vi "listen connection LV15.vi"(8 "Bool Refnum":refnum<vi>, 10 "service name":string="192.168.1.10") -> (1 "Numeric 2":i32, 2 "Boolean 3":bool, 3 "data out":string)   [LabVIEW 2020]
uses:
  Galobal variable_TI.vi
panel:
  out "length":i32
  out "String":string
  out "error out 3":errorcluster
  # "1,3.644,3.358,7.44,7.546"
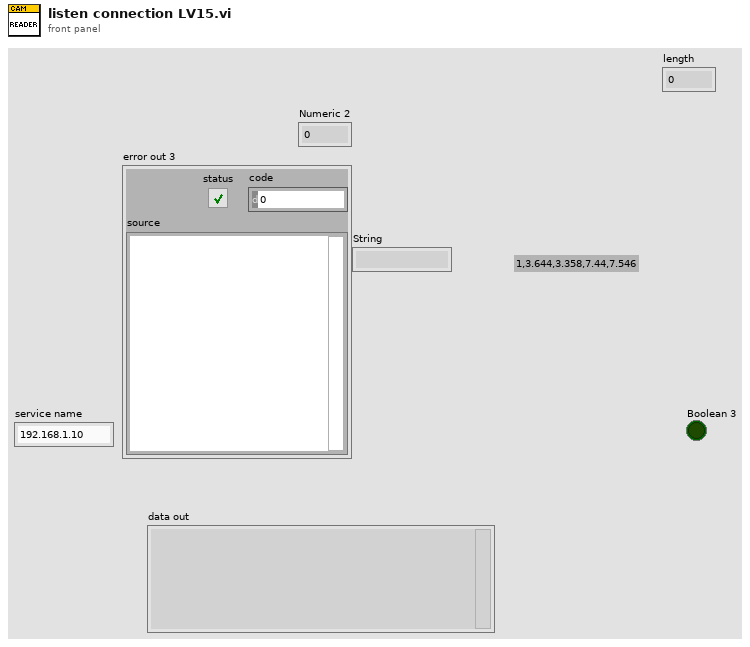
[diagram p1: front panel]
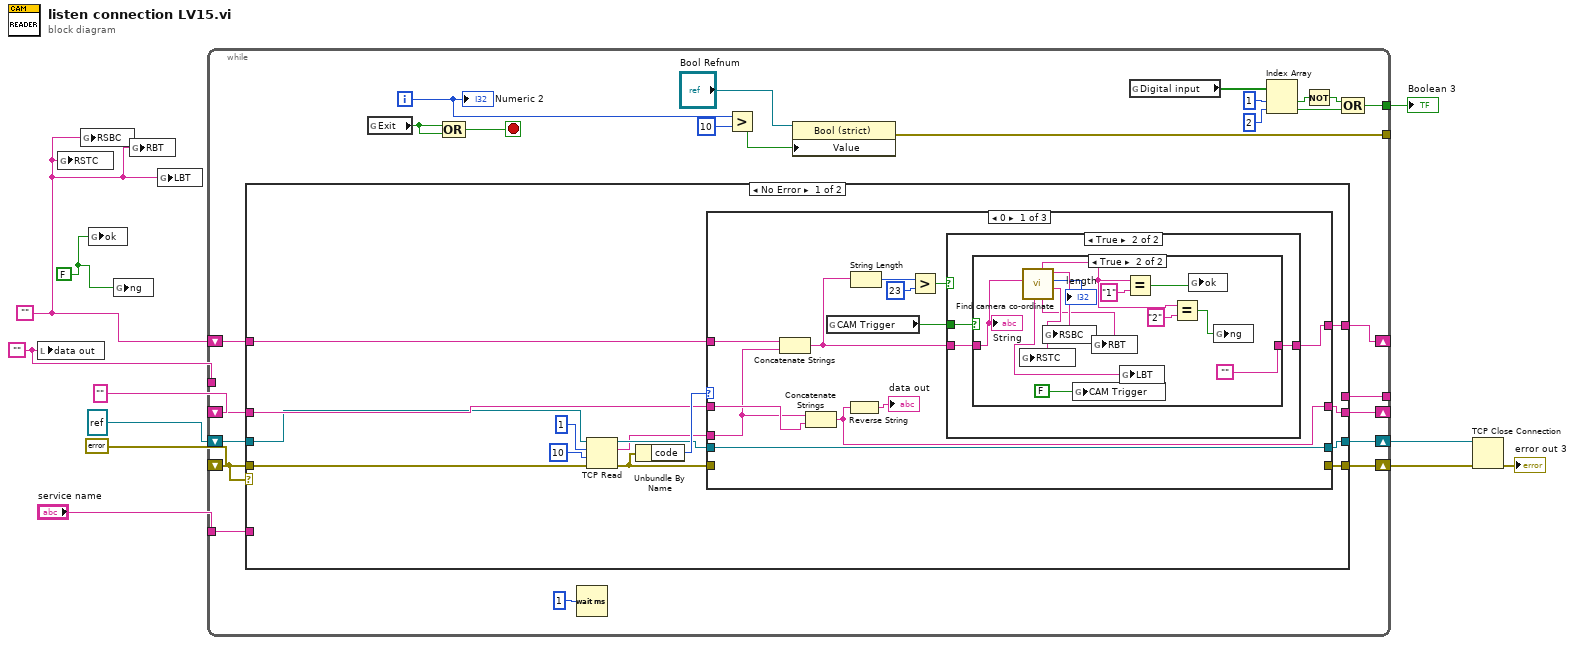
[diagram p0: block diagram]
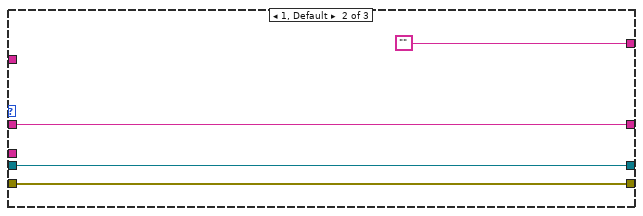
[diagram p4: hidden frame]
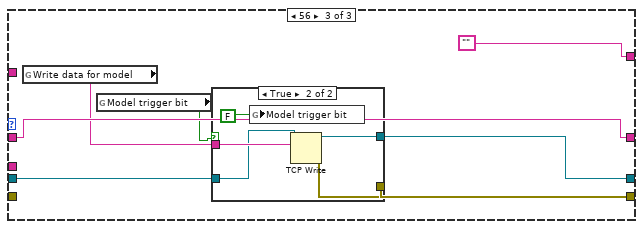
[diagram p5: hidden frame]
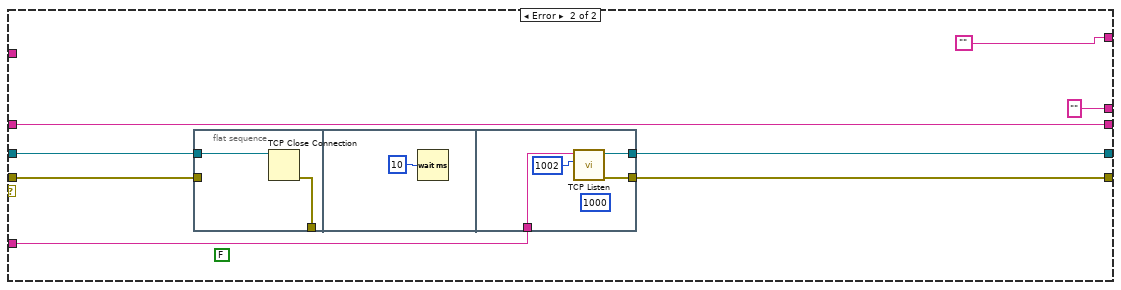
[diagram p7: hidden frame]
diagram:
  w1 = FALSE
  w2 = ""
  w3 = ""
  n1 = local write "data out"(w3) -> ()
  n2 = global write "Galobal variable_TI.vi" "RSTC"(w2) -> ()
  n3 = global write "Galobal variable_TI.vi" "RSBC"(w2) -> ()
  n4 = global write "Galobal variable_TI.vi" "ok"(w1) -> ()
  n5 = global write "Galobal variable_TI.vi" "ng"(w1) -> ()
  n6 = global write "Galobal variable_TI.vi" "RBT"(w2) -> ()
  n7 = global write "Galobal variable_TI.vi" "LBT"(w2) -> ()
  n8 = while {
    tunnel: [w34] -> _
    shift-right: [w36] -> w11
    shift-left: refnum<k5> refnum ("connection ID") -> [w33]
    shift-right: [w35] -> w10
    shift-left: errorcluster {"status"=FALSE, "code"=0, "source"=""} ("error out") -> [w32]
    tunnel: "service name" -> [w31]
    shift-right: [w21] -> _
    shift-left: "" -> [w30]
    tunnel: [w20] -> w4
    tunnel: w3 -> [_]
    shift-right: [w17] -> _
    shift-left: w2 -> [w18]
    tunnel: [w13] -> _
    i -> [w12]
    stop <- w28 stop-if-true
    n9 = case shown="No Error" w32 {
      tunnel: [w47 w101] -> w36
      tunnel: [w46 w100] -> w35
      tunnel: [_ "" ("data out")] -> w34
      tunnel: w33 -> [w38 w105]
      tunnel: w32 -> [w37 w104]
      tunnel: w31 -> [_ w103]
      tunnel: [w41 w102] -> w21
      tunnel: w30 -> [w43 w102]
      tunnel: w18 -> [w40 _]
      tunnel: [w39 ""] -> w17
      frame No Error {
        n10 = TCP Read(connection ID=w38, bytes to read=1, error in (no error)=w37, 9:10 ("timeout ms (25000)")) -> (connection ID out=w48:refnum<k5>, data out=w44:string, error out=w45:errorcluster)  [unwired: 1 in]
        n11 = Unbundle By Name(w45) -> ("code"=w49:i32)
        n12 = case shown="0" w49 {
          tunnel: w48 -> [w62 w83 w86]
          tunnel: [w62 w83 w88] -> w47
          tunnel: [_ w84 w87] -> w46
          tunnel: w45 -> [_ w84 _]
          tunnel: w44 -> [w53 _ _]
          tunnel: [w55 w82 w91] -> w41
          tunnel: w43 -> [w56 w82 w91]
          tunnel: w40 -> [w54 _ _]
          tunnel: [w52 "" ""] -> w39
          frame 0 {
            n13 = Concatenate Strings(w54, w53) -> (w51:string)
            n14 = Concatenate Strings(w53, w56) -> (w55:string)
            n15 = global read "Galobal variable_TI.vi" "CAM Trigger"() -> (w59:bool)
            n16 = Reverse String(1:w55) -> (0:→"data out":string)
            n17 = String Length(string=w51) -> (length=w61:i32)
            n18 = Greater?(x=w61, y=23) -> (0:w60:bool)
            n19 = case shown="True" w60 {
              tunnel: w59 -> [_ w66]
              tunnel: w51 -> [w63 w65]
              tunnel: [w63 w64] -> w52
              frame False {
              }
              frame True {
                n20 = case shown="True" w66 {
                  tunnel: w65 -> [w67 w74]
                  tunnel: [w67 ""] -> w64
                  frame False {
                  }
                  frame True {
                    n21 = call "Find camera co-ordinate.vi"("Read cam"=w74) -> ("RSTC"=w71:string, "length"=→"length":i32, "RSBC"=w72:string, "RBT"=w70:string, "ok/ng"=w73:string, "LBT"=w69:string)  [unwired: 5 in]
                    n22 = global write "Galobal variable_TI.vi" "RSTC"(w71) -> ()
                    n23 = global write "Galobal variable_TI.vi" "RSBC"(w72) -> ()
                    n24 = global write "Galobal variable_TI.vi" "CAM Trigger"(FALSE ("CAMERA TRIGGER")) -> ()
                    n25 = global write "Galobal variable_TI.vi" "RBT"(w70) -> ()
                    n26 = global write "Galobal variable_TI.vi" "LBT"(w69) -> ()
                    n27 = Equal?(x=w73, y="1") -> (x = y?=w77:bool)
                    n28 = Equal?(x=w73, y="2") -> (x = y?=w76:bool)
                    n29 = global write "Galobal variable_TI.vi" "ok"(w77) -> ()
                    n30 = global write "Galobal variable_TI.vi" "ng"(w76) -> ()
                    "String" <- w74
                  }
                }
              }
            }
          }
          frame 1, Default {
          }
          frame 56 {
            n31 = global read "Galobal variable_TI.vi" "Write data for model"() -> (w89:string)
            n32 = global read "Galobal variable_TI.vi" "Model trigger bit"() -> (w85:bool)
            n33 = case shown="True" w85 {
              tunnel: w89 -> [_ w97]
              tunnel: [w92 w96] -> w88
              tunnel: [_ w95] -> w87
              tunnel: w86 -> [w92 w94]
              frame False {
              }
              frame True {
                n34 = global write "Galobal variable_TI.vi" "Model trigger bit"(FALSE ("Model triger")) -> ()
                n35 = TCP Write(connection ID=w94, data in=w97) -> (connection ID out=w96:refnum<k5>, error out=w95:errorcluster)  [unwired: 2 in, 1 out]
              }
            }
          }
        }
      }
      frame Error {
        (unwired) FALSE
        n36 = flat-sequence {
          tunnel: w105 -> [w107]
          tunnel: w104 -> [_]
          tunnel: [w106] -> _
          tunnel: w103 -> [w111]
          tunnel: [w110] -> w101
          tunnel: [w109] -> w100
          frame #0 {
            n37 = TCP Close Connection(connection ID=w107) -> (error out=w106:errorcluster)  [unwired: 2 in, 1 out]
          }
          frame #1 {
            n38 = Wait (ms)(milliseconds to wait=u32 10) -> ()  [unwired: 1 out]
          }
          frame #2 {
            (unwired) 1000 ("timeout ms (wait forever: -1)")
            n39 = call <vilib>:"TCP Listen.vi"("port"=u16 1002, "service name"=w111) -> ("error out"=w109:errorcluster, "connection ID"=w110:refnum<k5>)  [unwired: 5 in, 3 out]
          }
        }
      }
    }
    n40 = global read "Galobal variable_TI.vi" "Exit"() -> (w19:bool)
    n41 = Compound Arithmetic op=OR(w19, w19) -> (w28:bool)
    n42 = Wait (ms)(milliseconds to wait=u32 1) -> ()  [unwired: 1 out]
    n43 = Greater?(x=w12, y=10) -> (0:w15:bool)
    n44 = property class="Bool (strict)"(reference="Bool Refnum", "Value"=w15) -> (error out=w13:errorcluster)  [unwired: 1 in, 1 out]
    n45 = global read "Galobal variable_TI.vi" "Digital input"() -> (w27:bool[])
    n46 = Index Array(array=w27, index #1=1 ("index"), index #2=2 ("index")) -> (element #1=w24:bool, element #2=w22:bool)
    n47 = Not(x=w24) -> (.not. x?=w23:bool)
    n48 = Compound Arithmetic op=OR(w23, w22) -> (w20:bool)
    "Numeric 2" <- w12
  }
  "Boolean 3" <- w4
  n49 = TCP Close Connection(connection ID=w11, error in (no error)=w10) -> (error out=→"error out 3":errorcluster)  [unwired: 1 in, 1 out]
